vi "Tracking_CloseFile.vi"(8 "error in":errorcluster, 11 "Tracking Data":T1) -> (0 "error out":errorcluster)   [LabVIEW 2017, in "ImageAcquisitionLibrary.lvlib"]
uses:
  ImageAcquisitionProgram/ImageAcquisitionLibrary/ImageAcquisitionLibrary.lvlib
  TrackingData.ctl
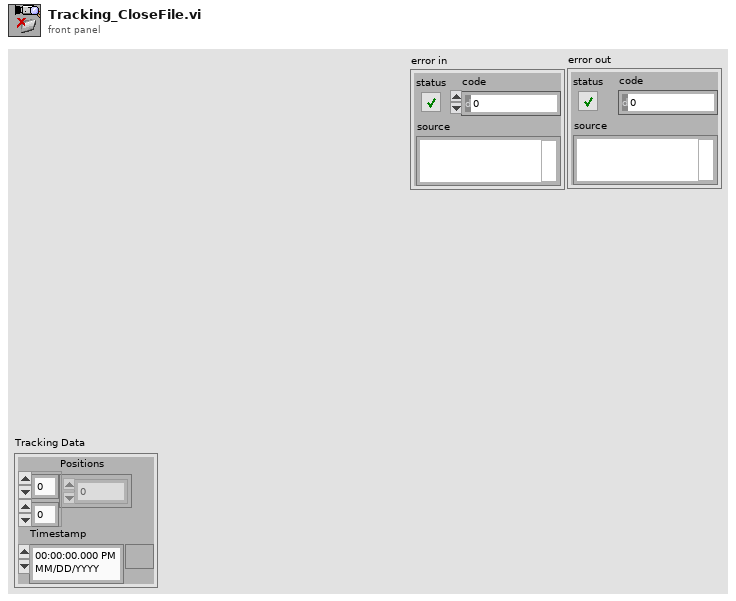
[diagram p1: front panel]
types:
  T1 = typedef "ImageAcquisitionLibrary.lvlib/TrackingData.ctl" = cluster{"Positions":dbl[][], "Timestamp":timestamp}
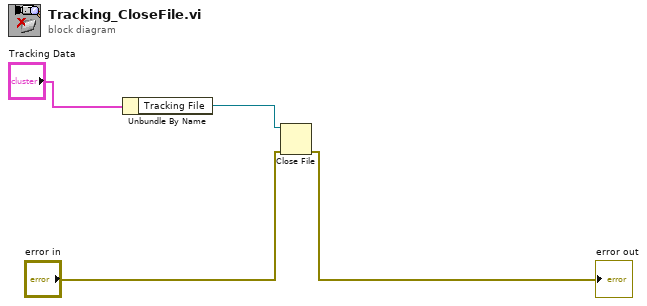
[diagram p0: block diagram]
diagram:
  n1 = Unbundle By Name("Tracking Data") -> ("Tracking File"=w3:refnum<file>)
  n2 = Close File(refnum=w3, error in="error in") -> (error out=→"error out":errorcluster)  [unwired: 1 out]
